vi "Actor Core.vi"(8 "error in":errorcluster, 11 "Test_Caller in":refnum<class "Test_Caller.lvclass">) -> (0 "error out":errorcluster, 3 "Actor out":refnum<class "Actor.lvclass">)   [LabVIEW 2025, in "Test_Caller.lvlib" / "Test_Caller.lvclass"]
doc: "<p>(<strong>Filename</strong>: <span class=\"dnl\">Actor Framework.lvlib:Actor.lvclass:Actor Core.vi</span>)</p>\n<p>Receives messages to the actor, reacts to them, and initiates any error handling that may shut the actor down.</p>\n<p>Descendant classes may override this VI to append parallel tasks for the actor to complete while it handles messages. Overrides use the <a href=\"nihelplauncher://docs/csh?context=lvcore_glang_udclass\">Call Parent Class Method</a> node.</p>"
uses:
  Test_Caller.lvclass
  C:/Program Files (x86)/National Instruments/LabVIEW 2025/vi.lib/ActorFramework/Actor/Actor.lvclass
  <vilib>/ActorFramework/Actor/Actor.lvclass
  Test_Nested/Test_Nested/Test_Nested.lvclass
  Test_Caller Messages/Update_UI Msg/Update_UI Msg.lvclass
  C:/Users/halstead_rideriver/Documents/Labview_Practice/ATM_Machine_Actor Framework/ATM_ACTORFW/Test_Nested/Test_Nested Messages/New Data Msg/New Data Msg.lvclass
  Test_Nested/Test_Nested/Test_Nested.lvclass/Test_Nested.ctl
  <vilib>/ActorFramework/Actor/Actor.lvclass/Actor.ctl
  <vilib>/ActorFramework/Message Enqueuer/Message Enqueuer.lvclass/Message Enqueuer.ctl
  Test_Caller.lvclass/Test_Caller.ctl
  <vilib>/ActorFramework/Message Enqueuer/Init from Existing Queue.vi
  <vilib>/ActorFramework/Message Enqueuer/Message Enqueuer.lvclass
  <vilib>/ActorFramework/Stop Msg/Stop Msg.lvclass
panel:
  out "Data received.":string
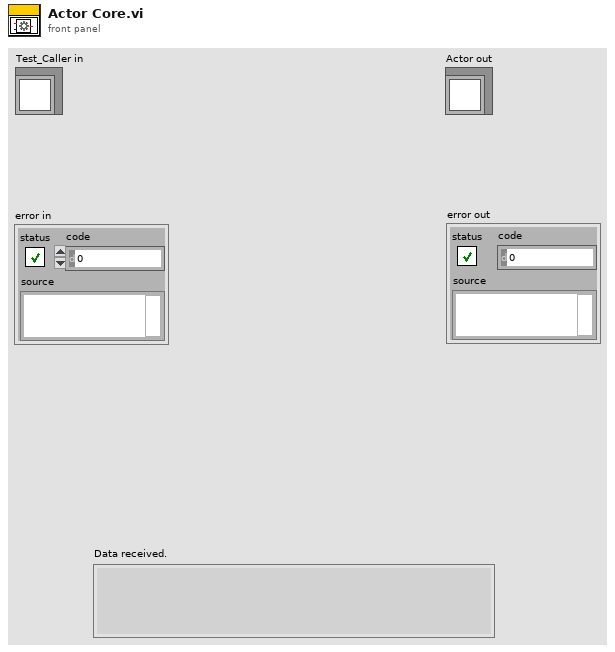
[diagram p1: front panel]
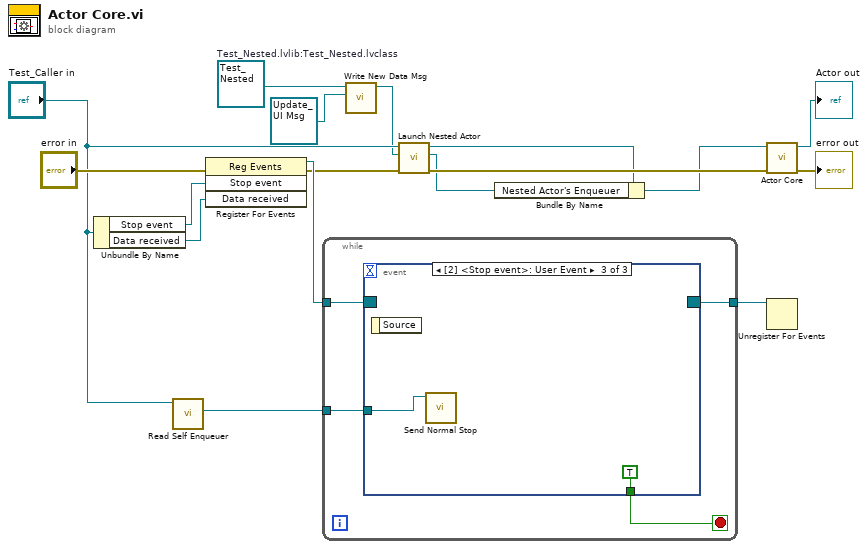
[diagram p0: block diagram]
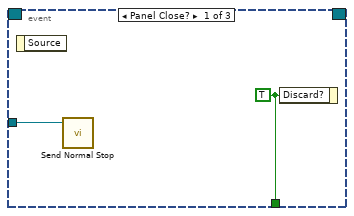
[diagram p2: hidden frame]
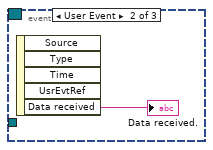
[diagram p3: hidden frame]
diagram:
  w9 = refnum<class "Test_Nested.lvclass"> refnum  # Test_Nested.lvlib:Test_Nested.lvclass
  n1 = Unbundle By Name("Test_Caller in") -> ("Stop event"=w13:refnum<user-event>, "Data received"=w12:refnum<user-event>)
  n2 = call <vilib>:"Read Self Enqueuer.vi"("Actor"="Test_Caller in") -> ("Self Enqueuer"=w10:refnum<class "Message Enqueuer.lvclass">)  [unwired: 10 in]
  n3 = register-events(error in="error in", w13, w12) -> (reference out=w14:refnum<event-registration>, error out=w6:errorcluster)  [unwired: 1 in]
  n4 = while {
    tunnel: w14 -> [w20]
    tunnel: [w19] -> w11
    tunnel: w10 -> [w18]
    stop <- w21 stop-if-true
    n5 = event shown="[2] <Stop event>: User Event" {
      selector: w20 -> [_ _ _]
      dyn-events: [_ _ _] -> w19
      timeout: _ -> [_ _ _]
      tunnel: [w23 _ TRUE ("Discard?")] -> w21
      tunnel: w18 -> [w22 _ w25]
      event Panel Close? {
        w23 = TRUE ("Discard?")
        n6 = event-data() -> ()  [unwired: 1 in, 1 out]
        n7 = call <vilib>:"Send Normal Stop.vi"("Message Enqueuer"=w22) -> ()  [unwired: 10 in, 1 out]
        n8 = event-data("Discard?"=w23) -> ()  [unwired: 1 in, 1 out]
      }
      event User Event {
        n9 = event-data() -> ("Data received"=→"Data received.":string)  [unwired: 1 in, 4 out]
      }
      event User Event {
        n10 = event-data() -> ()  [unwired: 1 in, 1 out]
        n11 = call <vilib>:"Send Normal Stop.vi"("Message Enqueuer"=w25) -> ()  [unwired: 10 in, 1 out]
      }
    }
  }
  n12 = call "Write New Data Msg.vi"("Test_Nested.lvlib:New Data Msg.lvclass"=refnum<class "Update_UI Msg.lvclass"> refnum ("Test_Caller.lvlib:Update_UI Msg.lvclass"), "Test_Nested in"=w9) -> ("Test_Nested out"=w4:refnum<class "Test_Nested.lvclass">)  [unwired: 9 in]
  n13 = call <vilib>:"Launch Nested Actor.vi"("error in (no error)"=w6, "Nested Actor"=w4, "Caller Actor in"="Test_Caller in") -> ("error out"=w5:errorcluster, "Nested Actor's Enqueuer"=w2:refnum<class "Message Enqueuer.lvclass">, "Caller Actor out"=w3:refnum<class "Test_Caller.lvclass">)  [unwired: 6 in]
  n14 = Bundle By Name(cluster=w3, "Nested Actor's Enqueuer"=w2) -> (w1:refnum<class "Test_Caller.lvclass">)
  n15 = call-parent "Actor Core.vi"("error in"=w5, "Actor in"=w1) -> ("error out"=→"error out":errorcluster, "Actor out"=→"Actor out":refnum<class "Actor.lvclass">)  [unwired: 8 in]
  n16 = Unregister For Events(event registration refnum=w11) -> ()  [unwired: 1 in, 1 out]
